vi "DeferPanelUpdate.vi"(8 "error in (no error)":errorcluster, 10 "Defer? (F)":bool, 11 "Tree_LVOOP__lava_lib_tree_class in":refnum<class "Tree Class.lvclass">) -> (0 "error out":errorcluster, 3 "Tree_LVOOP__lava_lib_tree_class out":refnum<class "Tree Class.lvclass">)   [LabVIEW 2012, in "Tree Tools.lvlib" / "Tree Class.lvclass"]
uses:
  Tree Class.lvclass
  Tree Class.lvclass/Tree Class.ctl
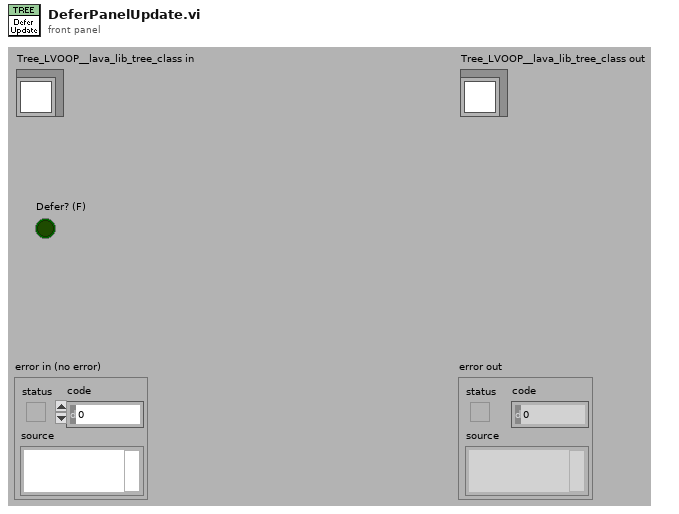
[diagram p1: front panel]
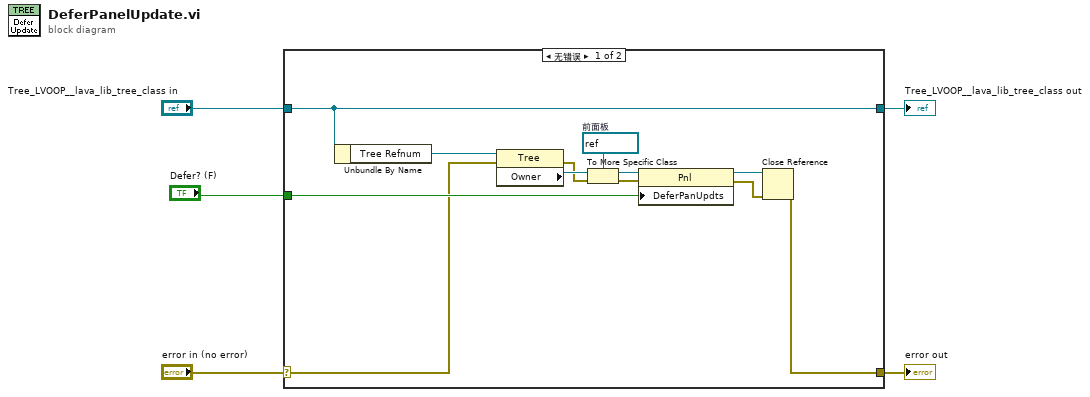
[diagram p0: block diagram]
diagram:
  n1 = case shown="无错误" "error in (no error)" {
    selector: "error in (no error)" -> [w9 w19]
    tunnel: [w6 w19] -> w4
    tunnel: [w17 w18] -> w2
    tunnel: "Tree_LVOOP__lava_lib_tree_class in" -> [w17 w18]
    tunnel: "Defer? (F)" -> [w12 _]
    frame No Error {
      w14 = refnum<vi> refnum  # 前面板
      n2 = Unbundle By Name(w17) -> ("Tree Refnum"=w13:refnum<vi>)
      n3 = property class="Tree"(reference=w13, error in=w9) -> (error out=w11:errorcluster, "Owner"=w16:refnum<vi>)  [unwired: 1 out]
      n4 = To More Specific Class(target class=w14, reference=w16, error in=w11) -> (specific class reference=w15:refnum<vi>, error out=w10:errorcluster)
      n5 = property class="Pnl"(reference=w15, error in=w10, "DeferPanUpdts"=w12) -> (reference out=w8:refnum<vi>, error out=w7:errorcluster)
      n6 = Close Reference(reference=w8, error in (no error)=w7) -> (error out=w6:errorcluster)
    }
    frame Error {
    }
  }
  "error out" <- w4
  "Tree_LVOOP__lava_lib_tree_class out" <- w2
